vi "Read CheesyVision.vi"(11 "Run?":bool) -> (2 "Direction":dbl, 3 "Done":bool)   [LabVIEW 2013]
panel:
  out "data out":string
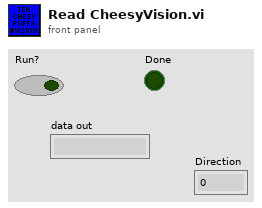
[diagram p1: front panel]
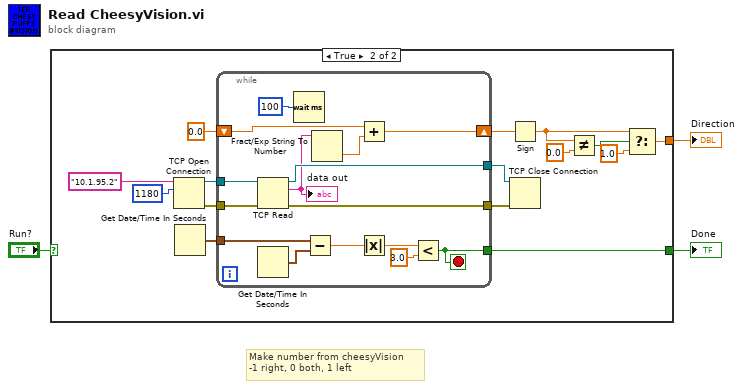
[diagram p0: block diagram]
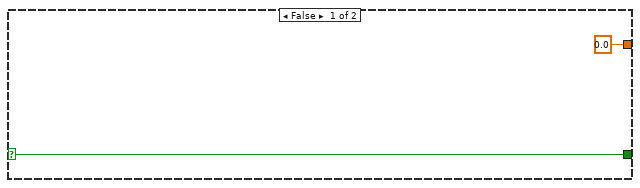
[diagram p2: hidden frame]
diagram:
  # "Make number from cheesyVision\n-1 right, 0 both, 1 left"
  n1 = case shown="True" "Run?" {
    selector: "Run?" -> [w5 _]
    tunnel: [w5 w13] -> w2
    tunnel: [0.0 ("f") w6] -> w1
    frame False {
    }
    frame True {
      n2 = TCP Open Connection(address="10.1.95.2", remote port or service name=u16 1180) -> (connection ID=w20:refnum<k5>, error out=w19:errorcluster)  [unwired: 3 in]
      n3 = Get Date/Time In Seconds() -> (seconds since 1Jan1904=w14:timestamp)
      n4 = while {
        tunnel: w20 -> [w34]
        tunnel: w19 -> [w33]
        tunnel: [w32] -> w16
        tunnel: [w31] -> w15
        tunnel: w14 -> [w30]
        tunnel: [w21] -> w13
        shift-right: [w23] -> w11
        shift-left: 0.0 -> [w22]
        stop <- w21 stop-if-true
        n5 = TCP Read(connection ID=w34, error in (no error)=w33) -> (connection ID out=w32:refnum<k5>, data out=w25:string, error out=w31:errorcluster)  [unwired: 3 in]
        "data out" <- w25
        n6 = Get Date/Time In Seconds() -> (seconds since 1Jan1904=w29:timestamp)
        n7 = Wait (ms)(milliseconds to wait=u32 100) -> ()  [unwired: 1 out]
        n8 = Subtract(x=w30, y=w29) -> (x-y=w28:dbl)
        n9 = Fract/Exp String To Number(string=w25) -> (number=w24:dbl)  [unwired: 3 in, 1 out]
        n10 = Add(x=w22, y=w24) -> (x+y=w23:dbl)
        n11 = Absolute Value(x=w28) -> (abs(x)=w27:dbl)
        n12 = Less?(x=w27, y=3.0) -> (x < y?=w21:bool)
      }
      n13 = Sign(1:w11) -> (0:w8:dbl)
      n14 = TCP Close Connection(connection ID=w16, error in (no error)=w15) -> ()  [unwired: 1 in, 2 out]
      n15 = Not Equal?(x=w8, y=0.0) -> (x != y?=w9:bool)
      n16 = Select(t=w8, s=w9, f=1.0) -> (s? t:f=w6:dbl)
    }
  }
  "Done" <- w2
  "Direction" <- w1
